vi "Step jsObject.vi"(8 "error in (no error)":errorcluster, 9 "Step Record (empty)":T1, 10 "Step jsObject Name (\"\")":string, 11 "Previous String (\"\")":string) -> (0 "error out":errorcluster, 2 "Step jsObject":string, 3 "STEP definition":string)   [LabVIEW 2011]
uses:
  Step Record.ctl
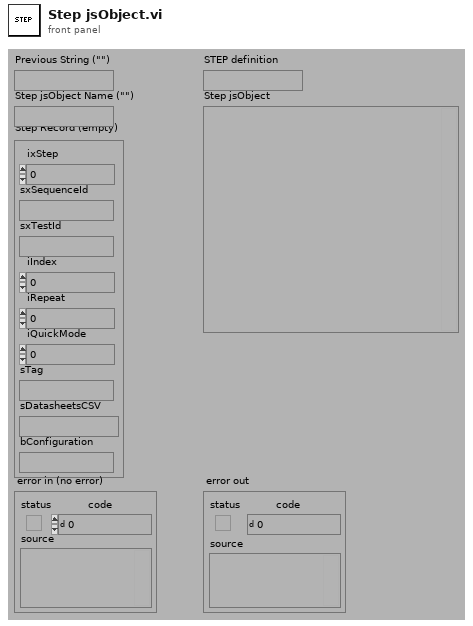
[diagram p1: front panel]
types:
  T1 = typedef "Step Record.ctl" = cluster{"ixStep":i32, "sxSequenceId":string, "sxTestId":string, "iIndex":i32, "iRepeat":i32, "iQuickMode":i32, "sTag":string, "sDatasheetsCSV":string, "bConfiguration":string}
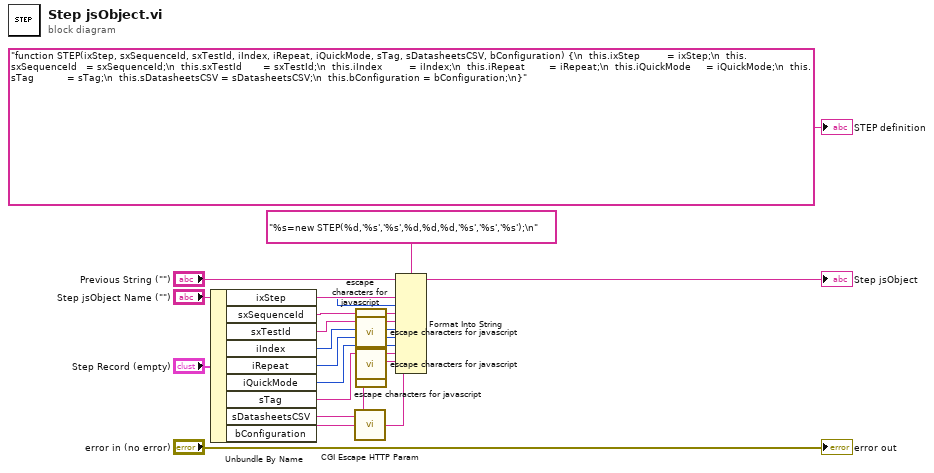
[diagram p0: block diagram]
diagram:
  n1 = Unbundle By Name("Step Record (empty)") -> ("ixStep"=w5:i32, "sxSequenceId"=w1:string, "sxTestId"=w11:string, "iIndex"=w10:i32, "iRepeat"=w9:i32, "iQuickMode"=w8:i32, "sTag"=w7:string, "sDatasheetsCSV"=w6:string, "bConfiguration"=w4:string)
  n2 = call "CGI Escape HTTP Param.vi"("string"=w4) -> ("url-encoded string"=w3:string)
  n3 = call "escape characters for javascript.vi"("String (\"\")"=w1) -> ("escaped String"=w2:string)  [unwired: 4 out]
  n4 = call "escape characters for javascript.vi"("String (\"\")"=w11) -> ("escaped String"=w15:string)  [unwired: 4 out]
  n5 = call "escape characters for javascript.vi"("String (\"\")"=w7) -> ("escaped String"=w14:string)  [unwired: 4 out]
  n6 = call "escape characters for javascript.vi"("String (\"\")"=w6) -> ("escaped String"=w13:string)  [unwired: 4 out]
  n7 = Format Into String(format string="%s=new STEP(%d,'%s','%s',%d,%d,%d,'%s','%s','%s');\n", initial string="Previous String (\"\")", "Step jsObject Name (\"\")", w5, w2, w15, w10, w9, w8, w14, w13, w3) -> (resulting string=→"Step jsObject":string)  [unwired: 1 in, 1 out]
  "error out" <- "error in (no error)"
  "STEP definition" <- "function STEP(ixStep, sxSequenceId, sxTestId, iIndex, iRepeat, iQuickMode, sTag, sDatasheetsCSV, bConfiguration) {\n  this.ixStep         = ixStep;\n  this.sxSequenceId   = sxSequenceId;\n  this.sxTestId       = sxTestId;\n  this.iIndex         = iIndex;\n  this.iRepeat        = iRepeat;\n  this.iQuickMode     = iQuickMode;\n  this.sTag           = sTag;\n  this.sDatasheetsCSV = sDatasheetsCSV;\n  this.bConfiguration = bConfiguration;\n}"
